vi "PH_PILS.set HV Greenlamp.vi"(0 "i ref in":refnum<vi>, 5 "error in (no error)":errorcluster) -> (14 "i ref out":refnum<vi>, 19 "error out":errorcluster)   [LabVIEW 2014, in "PH_PILS.lvlib"]
doc: "This VI switches flash lamp above door of the the HV-room in case of that the evacuation acqunoledgement is switched."
uses:
  PH_PILS.lvlib
  PH_Basics/PH_PP_Common/PH_PP_Common.PUs.ctl
  PH_Basics/PH_PP_Common/PH_PP_Common.PSU Tags.ctl
  PH_Devices/PH_Beckhoff_PPMA-Rods/PH_Beckhoff_PPMA-Rods.lvlib
  PH_Basics/PH_PP_Common/PH_PP_Common.lvlib
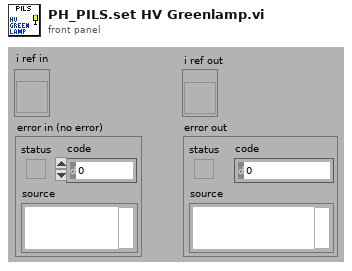
[diagram p1: front panel]
types:
  T1 = typedef "PH_PP_Common.lvlib/PH_PP_Common.PSU Tags.ctl" = enum16{"voltage-indicator", "peak-detect", "current", "voltage", "inihibit-indicator", "end-of-charge", "HV-on-indicator", "overtemperature", "interlock-indicator", "load-fault", "sum-fault", "HV-off-indicator", "DC-ok", "inhibit", "HV-on", "interlock", "reset", "Status", "Limits"}
  T2 = typedef "PH_PP_Common.lvlib/PH_PP_Common.PUs.ctl" = enum16{"no Info", "PA-19mm-1", "PA-19mm-2", "PA-45mm-PILC", "PA-45mm-MAIN", "MA-PU-1", "MA-PU-2", "MA-PU-3", "MA-PU-4", "MA-PU-5", "MA-PU-6", "MA-FR", "MA-PILC", "PA-45mm-DP"}
  T3 = typedef "PH_PILS.lvlib/PH_PILS.i attribute.ctl" = cluster{"Boolean":cluster{"GUI Ref":refnum<vi>, "Status":i32}[], "GUI Refs Exp. Shutters":cluster{"1":refnum<vi>, "2":refnum<vi>, "3":refnum<vi>, "4":refnum<vi>}, "Tristate2Run GUI Refs":refnum<vi>[], "EO-Likes":cluster{"GUI Ref":refnum<vi>, "Status":i32}[], "Operation Mode":cluster{"Operation Mode":T4, "GUI":cluster{"Ref State":refnum<vi>, "Ref":refnum<vi>}, "Servicemode":cluster{"Tagname":string, "Status":i32}, "Labormode":cluster{"Tagname":string, "Status":i32}, "Searchmode":cluster{"Tagname":string, "Status":i32}, "Shotmode":cluster{"Tagname":string, "Status":i32}}, "Submode":cluster{"Submode":T5, "GUI":cluster{"Ref State":refnum<vi>, "Ref":refnum<vi>}, "Submode":cluster{"Tagname":string, "Status":i32}}, "Experiment":cluster{"Experiment":enum16{"unknown", "intern", "4 (Z6)", "3", "2", "1"}, "GUI":cluster{"Ref State":refnum<vi>, "Ref":refnum<vi>}, "intern":cluster{"Tagname":string, "Status":i32}, "Exp 4":cluster{"Tagname":string, "Status":i32}, "Exp 3":cluster{"Tagname":string, "Status":i32}, "Exp 2":cluster{"Tagname":string, "Status":i32}, "Exp 1":cluster{"Tagname":string, "Status":i32}}, "TristateNormal":cluster{"GUI Ref":refnum<vi>, "Status":i32}[], "Door Tags":cluster{"GUI Ref":refnum<vi>, "Status":i32}[], "GUIlessTags":cluster{"Name":string, "Status":i32}[], "Beamline GUI Refs":refnum<vi>[], "Special Boolean":cluster{"GUI Ref":refnum<vi>, "Status":i32}[], "Laserpower":cluster{"GUI Ref":refnum<vi>, "Status":i32}[], "Shutter":cluster{"GUI Ref":refnum<vi>, "Status":i32}[], "Tristate EO Like":cluster{"GUI Ref":refnum<vi>, "Status":i32}[], "PP":cluster{"GUI Ref":refnum<vi>, "Status":i32, "Head Ref":refnum<vi>, "Slider Ref":refnum<vi>}[], "Switch Knobs":cluster{"GUI Ref":refnum<vi>, "Status":i32}[], "Latch Knob GUI Refs":refnum<vi>[], "FailureCounter":i32, "Enabled Status":cluster{"Laser":i32, "PreAmp":i32, "MainAmp":i32}, "Mercury":refnum<vi>, "Instance Rods":string, "Logfile":path, "Beckhoff-Instance Internal":string, "Beckhoff-Instance External":string, "Enabling Rights":cluster{"Name":string, "Password":string, "PA?":bool, "MA?":bool, "Exp?":bool}[]}
  T4 = typedef "PH_PILS.lvlib/PH_PILS.Operation Mode.ctl" = enum16{"unknown", "Service", "Labor", "Search", "Shot"}
  T5 = typedef "PH_PILS.lvlib/PH_PILS.Submode.ctl" = enum16{"unknown", "HV-Normal", "HV-Test"}
  T6 = cluster{"GUI Ref":refnum<vi>, "Status":i32, "Head Ref":refnum<vi>, "Slider Ref":refnum<vi>}[]
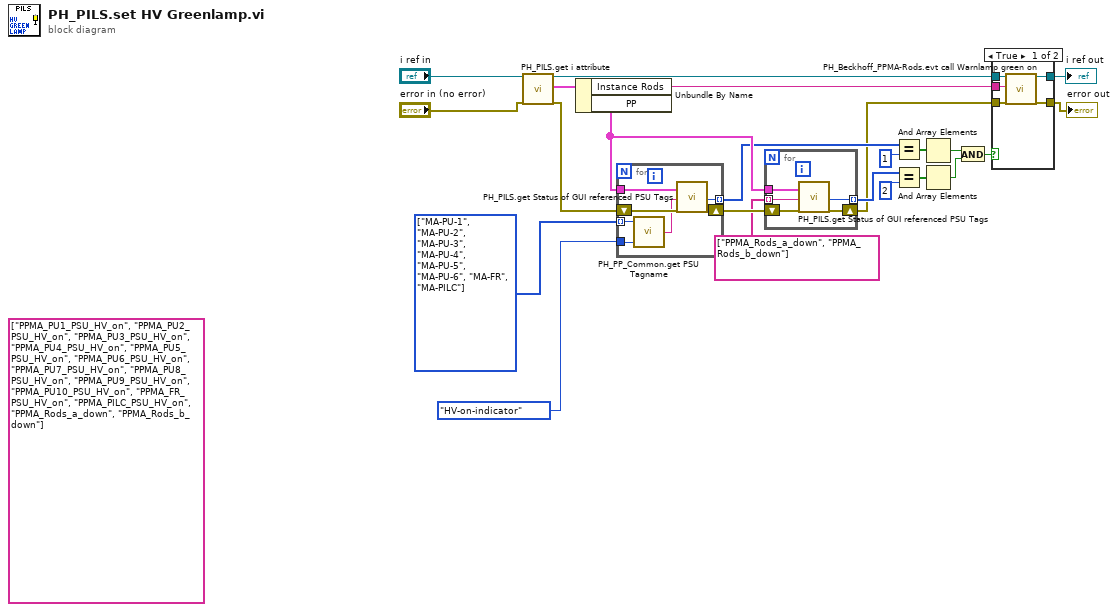
[diagram p0: block diagram]
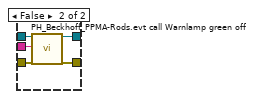
[diagram p2: hidden frame]
diagram:
  w2 = T2[] [enum."MA-PU-1", enum."MA-PU-2", enum."MA-PU-3", enum."MA-PU-4", enum."MA-PU-5", enum."MA-PU-6", enum."MA-FR", enum."MA-PILC"] items=["no Info", "PA-19mm-1", "PA-19mm-2", "PA-45mm-PILC", "PA-45mm-MAIN", "MA-PU-1", "MA-PU-2", "MA-PU-3", "MA-PU-4", "MA-PU-5", "MA-PU-6", "MA-FR", "MA-PILC", "PA-45mm-DP"]
  (unwired) string[] ["PPMA_PU1_PSU_HV_on", "PPMA_PU2_PSU_HV_on", "PPMA_PU3_PSU_HV_on", "PPMA_PU4_PSU_HV_on", "PPMA_PU5_PSU_HV_on", "PPMA_PU6_PSU_HV_on", "PPMA_PU7_PSU_HV_on", "PPMA_PU8_PSU_HV_on", "PPMA_PU9_PSU_HV_on", "PPMA_PU10_PSU_HV_on", "PPMA_FR_PSU_HV_on", "PPMA_PILC_PSU_HV_on", "PPMA_Rods_a_down", "PPMA_Rods_b_down"]
  n1 = call "PH_PILS.get i attribute.vi"("i ref in"="i ref in", "error in (no error)"="error in (no error)") -> ("i ref out"=w5:refnum<vi>, "i attribute"=w23:T3, "error out"=w15:errorcluster)  [unwired: 15 in]
  n2 = Unbundle By Name(w23) -> ("Instance Rods"=w3:string, "PP"=w17:T6)
  n3 = for {
    tunnel: w17 -> [w27]
    shift-right: [w29] -> w18
    shift-left: w15 -> [w30]
    tunnel: [w28] -> w14 mode=indexing
    tunnel: w2 -> [w26] mode=indexing
    tunnel: PH_PP_Common.PSU_Tags."HV-on-indicator" ("PSU Tag") -> [w25]
    n4 = call "PH_PP_Common.get PSU Tagname.vi"("PSU Tag"=w25, "PU"=w26) -> ("PSU Tagname"=w24:string)  [unwired: 1 in]
    n5 = call "PH_PILS.get Status of GUI referenced PSU Tags.vi"("PP Tag"=w27, "Tagname"=w24, "error in"=w30) -> ("Status"=w28:i32, "error out"=w29:errorcluster)  [unwired: 11 in, 4 out]
  }
  n6 = for {
    tunnel: w17 -> [w31]
    shift-right: [w34] -> w4
    shift-left: w18 -> [w35]
    tunnel: string[] ["PPMA_Rods_a_down", "PPMA_Rods_b_down"] -> [w32] mode=indexing
    tunnel: [w33] -> w11 mode=indexing
    n7 = call "PH_PILS.get Status of GUI referenced PSU Tags.vi"("PP Tag"=w31, "Tagname"=w32, "error in"=w35) -> ("Status"=w33:i32, "error out"=w34:errorcluster)  [unwired: 11 in, 4 out]
  }
  n8 = Equal?(x=w14, y=1 ("Status")) -> (x = y?=w10:bool[])
  n9 = Equal?(x=w11, y=2 ("Status")) -> (x = y?=w9:bool[])
  n10 = And Array Elements(Boolean array=w10) -> (logical AND=w8:bool)
  n11 = And Array Elements(Boolean array=w9) -> (logical AND=w7:bool)
  n12 = And(x=w8, y=w7) -> (x .and. y?=w6:bool)
  n13 = case shown="True" w6 {
    tunnel: [w40 w45] -> w20
    tunnel: [w39 w44] -> w19
    tunnel: w3 -> [w36 w41]
    tunnel: w5 -> [w38 w43]
    tunnel: w4 -> [w37 w42]
    frame True {
      n14 = call "PH_Beckhoff_PPMA-Rods.evt call Warnlamp green on.vi"("i ref in"=w38, "Instance name"=w36, "error in"=w37) -> ("i ref out"=w39:refnum<vi>, "error out"=w40:errorcluster)  [unwired: 15 in]
    }
    frame False {
      n15 = call "PH_Beckhoff_PPMA-Rods.evt call Warnlamp green off.vi"("i ref in"=w43, "Instance name"=w41, "error in"=w42) -> ("i ref out"=w44:refnum<vi>, "error out"=w45:errorcluster)  [unwired: 15 in]
    }
  }
  "i ref out" <- w19
  "error out" <- w20
